vi "test_SegmenterDL100224ThreeD.vi"() -> ()   [LabVIEW 2010, in "SegmenterDL100224ThreeD.lvclass"]
uses:
  SegmenterDL100224ThreeD.lvclass
  common/classes/ImageCollection/ImageCollection/ImageCollection.lvclass
  common/clusters/plugin_specification.ctl
  GenericSegmenter/GenericSegmenter/centroid_cluster.ctl
  <vilib>/vision/Image Controls.llb/IMAQ Image.ctl
  GenericSegmenter/GenericSegmenter/GenericSegmenter.lvclass
  common/classes/GenericComponent/GenericComponent/GenericComponent.lvclass
  common/classes/ImageCollection/ImageCollection/add_mode_enum.ctl
  common/classes/Image/Image/Image.lvclass
panel:
  in  "overlay centroids?":bool
  in  "overlay ROIs?":bool
  out "segmented image":T1(plugin-control)
  in  "segmentButton":bool
  in  "frame":i32(slide) scale=1.0..100.0
  out "original image":T1(plugin-control)
  in  "loadButton":bool
  in  "stopButton":bool
  in  "createButton":bool
  in  "configuration":string(combo)
  # "Test for Segmenter Classes"
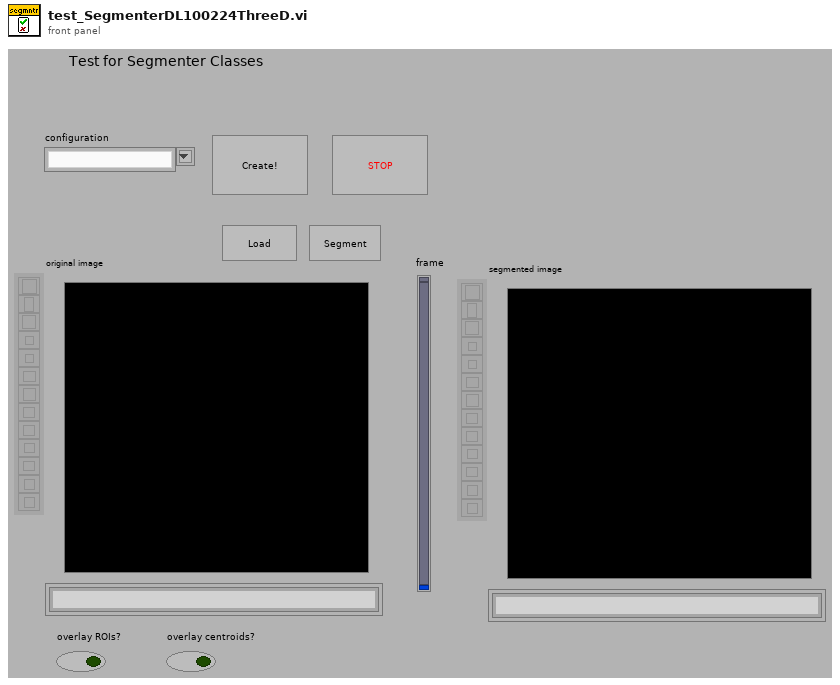
[diagram p1: front panel]
types:
  T1 = typedef "IMAQ Image.ctl" = refnum<image>
  T2 = typedef "GenericSegmenter.lvclass/centroid_cluster.ctl" = cluster{"x":i32, "y":i32, "z":i32, "number of pixels":i32}
  T3 = typedef "plugin_specification.ctl" = cluster{"class path":string, "configuration":string, "label":string, "settings name":string}
  T4 = cluster{"Left":i32, "Top":i32, "Right":i32, "Bottom":i32}
  T5 = typedef "Image Type" = u32
  T6 = typedef "ImageCollection.lvclass/add_mode_enum.ctl" = enum16{"instance", "copy"}
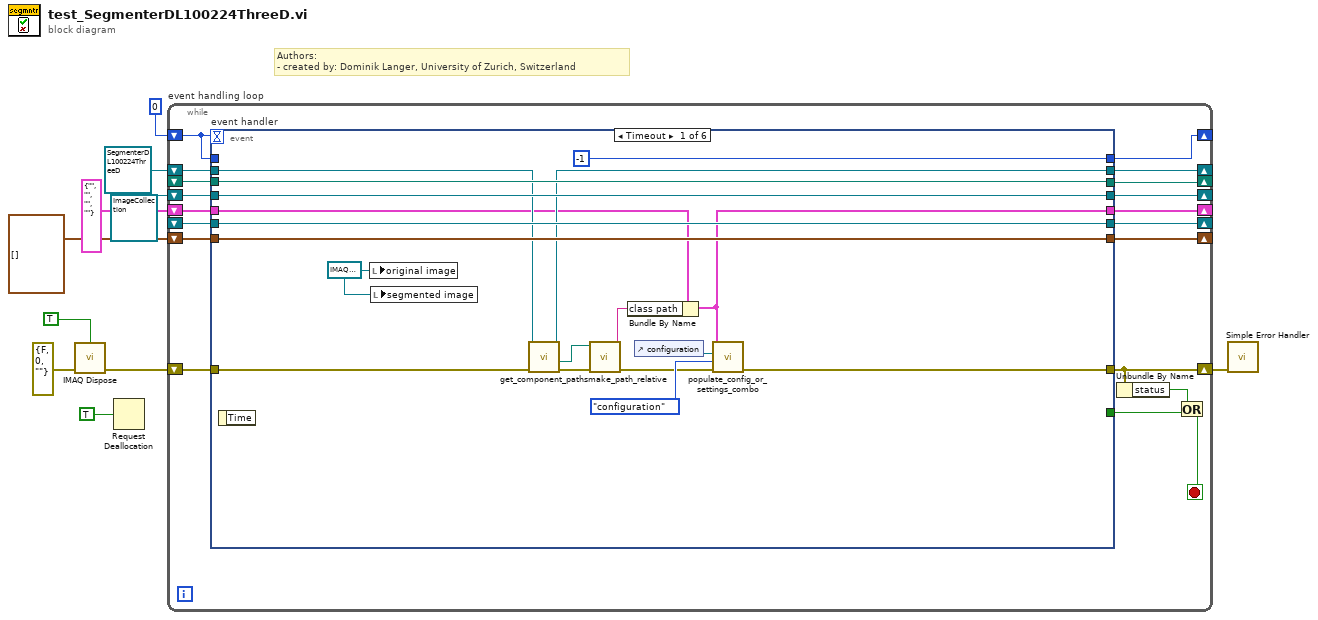
[diagram p0: block diagram]
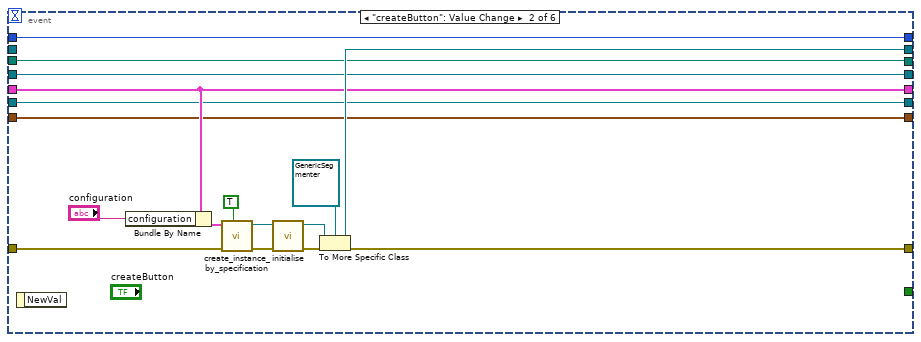
[diagram p2: hidden frame]
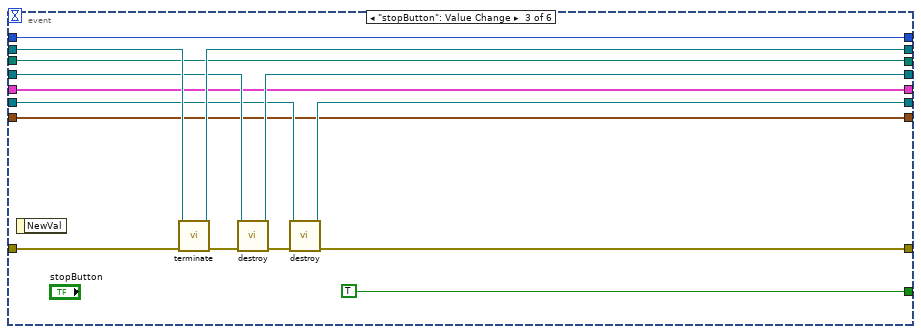
[diagram p3: hidden frame]
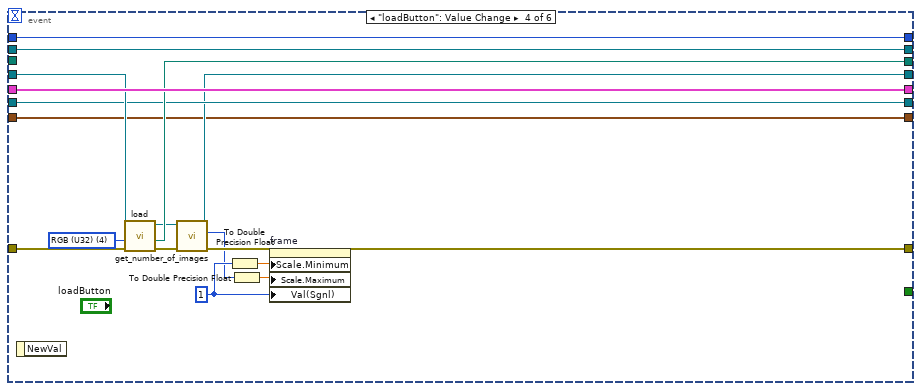
[diagram p4: hidden frame]
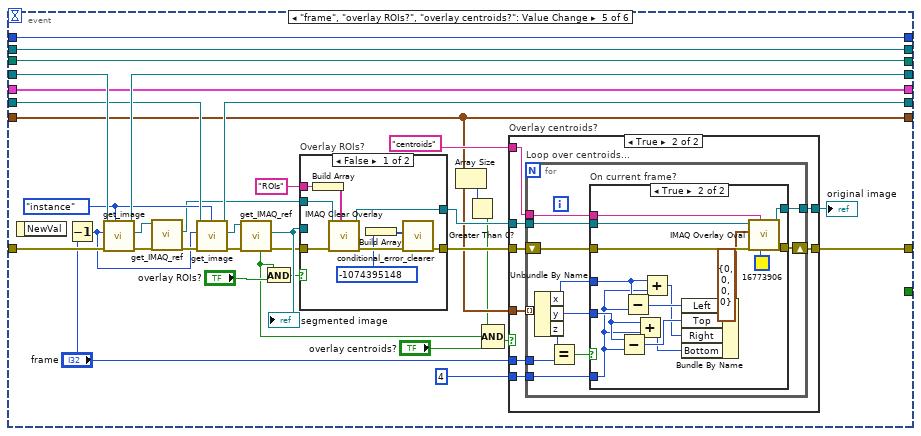
[diagram p5: hidden frame]
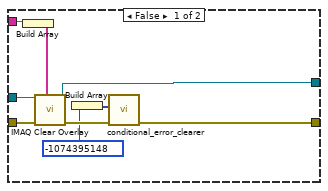
[diagram p6: hidden frame]
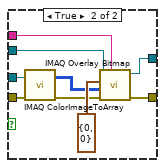
[diagram p8: hidden frame]
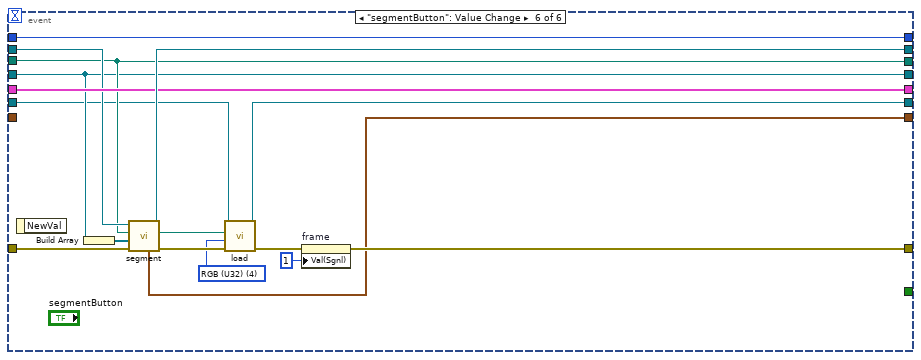
[diagram p9: hidden frame]
diagram:
  # "Authors: \n- created by: Dominik Langer, University of Zurich, Switzerland"
  n1 = call "IMAQ Dispose"("All Images? (No)"=TRUE, "error in (no error)"=errorcluster {"status"=FALSE, "code"=0, "source"=""} ("error out")) -> ("error out"=w4:errorcluster)  [unwired: 4 in]
  n2 = Request Deallocation(TRUE ("flag")) -> ()
  n3 = while "event handling loop" {
    shift-right: [w11] -> w10
    shift-left: w4 -> [w29]
    shift-right: [w25] -> _
    shift-left: refnum<class "SegmenterDL100224ThreeD.lvclass"> refnum ("SegmenterDL100224ThreeD.lvclass") -> [w24]
    shift-right: [w22] -> _
    shift-left: refnum<class "ImageCollection.lvclass"> refnum ("ImageCollection.lvclass") -> [w23]
    shift-right: [w20] -> _
    shift-left: T3 {"class path"="", "configuration"="", "label"="", "settings name"=""} ("component specification") -> [w21]
    shift-right: [w19] -> _
    shift-left: _ -> [w18]
    shift-right: [w16] -> _
    shift-left: 0 -> [w17]
    shift-right: [w15] -> _
    shift-left: _ -> [w14]
    shift-right: [w12] -> _
    shift-left: T2[] [] -> [w13]
    stop <- w26 stop-if-true
    n4 = event "event handler" shown="[0] Timeout" {
      selector: _ -> [_ _ _ _ _ _]
      dyn-events: _ -> [_ _ _ _ _ _]
      timeout: w17 -> [_ _ _ _ _ _]
      tunnel: w29 -> [w36 w64 w78 w92 w131 w211]
      tunnel: [_ _ TRUE _ _ _] -> w27
      tunnel: [w33 w55 w76 w97 w132 w213] -> w25
      tunnel: w24 -> [w34 _ w77 w97 w132 w210]
      tunnel: [w47 w54 w73 w85 w129 w206] -> w22
      tunnel: w23 -> [w47 w54 w74 w91 w130 w206]
      tunnel: w21 -> [w31 w53 w72 w96 w126 w212]
      tunnel: [w30 w53 w72 w96 w126 w212] -> w20
      tunnel: [w46 w51 w71 w94 w125 w209] -> w19
      tunnel: w18 -> [w46 w51 w71 _ w125 w209]
      tunnel: [-1 w50 w70 w95 w124 w208] -> w16
      tunnel: w17 -> [_ w50 w70 w95 w124 w208]
      tunnel: [w43 w49 w68 w89 w122 w204] -> w15
      tunnel: w14 -> [w43 w49 w69 w89 w123 w203]
      tunnel: w13 -> [w42 w48 w65 w80 w103 _]
      tunnel: [w42 w48 w65 w80 w103 w197] -> w12
      tunnel: [w37 w58 w66 w93 w109 w198] -> w11
      event Timeout {
        w44 = T1 refnum ("original image")
        n5 = event-data() -> ()  [unwired: 1 in, 1 out]
        n6 = local write "original image"(w44) -> ()
        n7 = local write "segmented image"(w44) -> ()
        n8 = call-dynamic "get_component_paths.vi"("error in (no error)"=w36, "GenericComponent in"=w34) -> ("error out"=w35:errorcluster, "component class path"=w32:path, "GenericComponent out"=w33:refnum<class "GenericSegmenter.lvclass">)  [unwired: 4 in, 3 out]
        n9 = call "make_path_relative.vi"("error in (no error)"=w35, "absolute path"=w32) -> ("error out"=w39:errorcluster, "relative path"=w38:string)  [unwired: 8 in]
        n10 = Bundle By Name(cluster=w31, "class path"=w38) -> (w30:T3)
        n11 = control-ref of="configuration"() -> (w40:refnum<vi>)
        n12 = call "populate_config_or_settings_combo.vi"("error in (no error)"=w39, "type"=enum16{"configuration", "settings"}."configuration", "combo-box reference"=w40, "plug-in specification"=w30) -> ("error out"=w37:errorcluster)  [unwired: 7 in]
      }
      event "createButton": Value Change {
        n13 = event-data() -> ()  [unwired: 1 in, 1 out]
        n14 = Bundle By Name(cluster=w53, "configuration"="configuration") -> (w62:T3)
        n15 = call "create_instance_by_specification.vi"("call constructor?"=TRUE, "error in (no error)"=w64, "component specification"=w62) -> ("error out"=w61:errorcluster, "GenericPlugin out"=w60:refnum<class "GenericComponent.lvclass">)  [unwired: 6 in, 1 out]
        n16 = call-dynamic "initialise.vi"("error in (no error)"=w61, "GenericPlugin in"=w60) -> ("error out"=w59:errorcluster, "GenericPlugin out"=w57:refnum<class "GenericComponent.lvclass">)  [unwired: 8 in]
        n17 = To More Specific Class(target class=refnum<class "GenericSegmenter.lvclass"> refnum ("GenericSegmenter.lvclass"), reference=w57, error in=w59) -> (specific class reference=w55:refnum<class "GenericSegmenter.lvclass">, error out=w58:errorcluster)
      }
      event "stopButton": Value Change {
        n18 = event-data() -> ()  [unwired: 1 in, 1 out]
        n19 = call-dynamic "terminate.vi"("error in (no error)"=w78, "GenericPlugin in"=w77) -> ("error out"=w75:errorcluster, "GenericPlugin out"=w76:refnum<class "GenericSegmenter.lvclass">)  [unwired: 8 in]
        n20 = call-dynamic "destroy.vi"("error in (no error)"=w75, "ImageCollection in"=w74) -> ("error out"=w67:errorcluster, "ImageCollection out"=w73:refnum<class "ImageCollection.lvclass">)  [unwired: 8 in]
        n21 = call-dynamic "destroy.vi"("error in (no error)"=w67, "ImageCollection in"=w69) -> ("error out"=w66:errorcluster, "ImageCollection out"=w68:refnum<class "ImageCollection.lvclass">)  [unwired: 8 in]
      }
      event "loadButton": Value Change {
        w90 = T5 4 items=["Grayscale (U8)", "Grayscale (I16)", "Grayscale (SGL)", "Complex (CSG)", "RGB (U32)", "HSL (U32)", "RGB (U64)", "Grayscale (U16)"] ("Image Type")
        w83 = 1 ("Value (Signaling)")
        n22 = event-data() -> ()  [unwired: 1 in, 1 out]
        n23 = call "load.vi"("error in (no error)"=w92, "Image Type"=w90, "ImageCollection in"=w91) -> ("error out"=w88:errorcluster, "path out"=w94:path, "ImageCollection out"=w86:refnum<class "ImageCollection.lvclass">)  [unwired: 4 in, 2 out]
        n24 = call-dynamic "get_number_of_images.vi"("error in (no error)"=w88, "ImageCollection in"=w86) -> ("error out"=w87:errorcluster, "size"=w82:i32, "ImageCollection out"=w85:refnum<class "ImageCollection.lvclass">)  [unwired: 7 in]
        n25 = To Double Precision Float(number=w83) -> (double precision float=w84:dbl)
        n26 = To Double Precision Float(number=w82) -> (double precision float=w81:dbl)
        n27 = property on="frame" class="Slide (strict)"(error in=w87, "Scale.Minimum"=w84, "Scale.Maximum"=w81, "Val(Sgnl)"=w83) -> (error out=w93:errorcluster)  [unwired: 1 in, 1 out]
      }
      event "frame", "overlay ROIs?", "overlay centroids?": Value Change {
        w119 = add_mode_enum."instance" ("get image as...")
        n28 = event-data() -> ()  [unwired: 1 in, 1 out]
        n29 = Decrement(x="frame") -> (x-1=w118:i32)
        n30 = call-dynamic "get_image.vi"("get image as..."=w119, "error in (no error)"=w131, "index"=w118, "ImageCollection in"=w130) -> ("error out"=w128:errorcluster, "Image.lvclass"=w127:refnum<class "Image.lvclass">, "ImageCollection out"=w129:refnum<class "ImageCollection.lvclass">)  [unwired: 5 in]
        n31 = call-dynamic "get_IMAQ_ref.vi"("error in (no error)"=w128, "Image.lvclass in"=w127) -> ("error out"=w121:errorcluster, "Image"=w116:T1)  [unwired: 5 in, 3 out]
        n32 = call-dynamic "get_image.vi"("get image as..."=w119, "error in (no error)"=w121, "index"=w118, "ImageCollection in"=w123) -> ("error out"=w117:errorcluster, "Image.lvclass"=w120:refnum<class "Image.lvclass">, "ImageCollection out"=w122:refnum<class "ImageCollection.lvclass">)  [unwired: 5 in]
        n33 = call-dynamic "get_IMAQ_ref.vi"("error in (no error)"=w117, "Image.lvclass in"=w120) -> ("error out"=w114:errorcluster, "Image"=w115:T1, "not empty?"=w100:bool)  [unwired: 5 in, 2 out]
        "segmented image" <- w115
        n34 = And(x=w100, y="overlay ROIs?") -> (x .and. y?=w112:bool)
        n35 = case "Overlay ROIs?" shown="False" w112 {
          tunnel: [w185 w196] -> w108
          tunnel: w116 -> [w186 w195]
          tunnel: w115 -> [_ w191]
          tunnel: w114 -> [w187 w192]
          tunnel: [w181 w193] -> w110
          tunnel: "ROIs" ("Group") -> [w184 w188]
          frame False {
            n36 = Build Array(w184) -> (w183:string[])
            n37 = call "IMAQ Clear Overlay"("Groups"=w183, "error in (no error)"=w187, "Image"=w186) -> ("error out"=w182:errorcluster, "Image Out"=w185:T1)  [unwired: 7 in]
            n38 = Build Array(-1074395148 ("error code")) -> (w180:i32[])
            n39 = call "conditional_error_clearer.vi"("error in (no error)"=w182, "array of clearable error codes"=w180) -> ("error out"=w181:errorcluster)  [unwired: 9 in]
          }
          frame True {
            n40 = call "IMAQ ColorImageToArray"("Image"=w191, "error in (no error)"=w192) -> ("Image Pixels (U32)"=w190:u32[][], "error out"=w189:errorcluster)  [unwired: 2 in, 1 out]
            n41 = call "IMAQ Overlay Bitmap"("Group"=w188, "error in (no error)"=w189, "Bitmap"=w190, "Top Left Point"=cluster{"X":i32, "Y":i32} {"X"=0, "Y"=0}, "Image"=w195) -> ("error out"=w193:errorcluster, "Image Out"=w196:T1)  [unwired: 5 in]
          }
        }
        n42 = Array Size(array=w103) -> (size(s)=w102:i32)
        n43 = Greater Than 0?(x=w102) -> (x > 0?=w98:bool)
        n44 = Compound Arithmetic op=AND(w98, w100, "overlay centroids?") -> (w99:bool)
        n45 = case "Overlay centroids?" shown="True" w99 {
          tunnel: w110 -> [w138 w149]
          tunnel: [w137 w148] -> w109
          tunnel: w103 -> [_ w147]
          tunnel: w108 -> [w134 w146]
          tunnel: "centroids" ("Group") -> [w136 w144]
          tunnel: [w133 w145] -> w106
          tunnel: "frame" -> [_ w143]
          tunnel: 4 -> [_ w142]
          frame False {
            n46 = Build Array(w136) -> (w135:string[])
            n47 = call "IMAQ Clear Overlay"("Groups"=w135, "error in (no error)"=w138, "Image"=w134) -> ("error out"=w141:errorcluster, "Image Out"=w133:T1)  [unwired: 7 in]
            n48 = Build Array(-1074395148 ("error code")) -> (w140:i32[])
            n49 = call "conditional_error_clearer.vi"("error in (no error)"=w141, "array of clearable error codes"=w140) -> ("error out"=w137:errorcluster)  [unwired: 9 in]
          }
          frame True {
            n50 = for "Loop over centroids..." {
              shift-right: [w158] -> w148
              shift-left: w149 -> [w160]
              tunnel: w147 -> [w161] mode=indexing
              tunnel: w146 -> [w159]
              tunnel: [w157] -> w145
              tunnel: w144 -> [w156]
              tunnel: w143 -> [w155]
              tunnel: w142 -> [w150]
              n51 = Unbundle By Name(w161) -> ("x"=w152:i32, "y"=w151:i32, "z"=w154:i32)
              n52 = Equal?(x=w154, y=w155) -> (x = y?=w153:bool)
              n53 = case "On current frame?" shown="True" w153 {
                tunnel: w160 -> [w162 w178]
                tunnel: w159 -> [w163 w177]
                tunnel: [w162 w176] -> w158
                tunnel: [w163 w175] -> w157
                tunnel: w156 -> [_ w174]
                tunnel: w152 -> [_ w171]
                tunnel: w151 -> [_ w172]
                tunnel: w150 -> [_ w170]
                frame False {
                }
                frame True {
                  n54 = Subtract(x=w172, y=w170) -> (x-y=w167:i32)
                  n55 = Subtract(x=w171, y=w170) -> (x-y=w168:i32)
                  n56 = Add(x=w172, y=w170) -> (x+y=w165:i32)
                  n57 = Add(x=w171, y=w170) -> (x+y=w166:i32)
                  n58 = Bundle By Name(cluster=T4 {"Left"=0, "Top"=0, "Right"=0, "Bottom"=0} ("Bounding Rectangle"), "Left"=w168, "Top"=w167, "Right"=w166, "Bottom"=w165) -> (w164:T4)
                  n59 = call "IMAQ Overlay Oval"("Color"=u32 16773906, "Group"=w174, "error in (no error)"=w178, "Bounding Rectangle"=w164, "Image"=w177) -> ("error out"=w176:errorcluster, "Image Out"=w175:T1)  [unwired: 5 in]
                }
              }
            }
          }
        }
        "original image" <- w106
      }
      event "segmentButton": Value Change {
        w201 = T5 4 items=["Grayscale (U8)", "Grayscale (I16)", "Grayscale (SGL)", "Complex (CSG)", "RGB (U32)", "HSL (U32)", "RGB (U64)", "Grayscale (U16)"] ("Image Type")
        n60 = event-data() -> ()  [unwired: 1 in, 1 out]
        n61 = Build Array(w206) -> (w207:refnum<class "ImageCollection.lvclass">[])
        n62 = call-dynamic "segment.vi"("error in (no error)"=w211, "ImageCollection in"=w207, "image file path"=w209, "GenericSegmenter in"=w210) -> ("error out"=w205:errorcluster, "segmented image path out"=w202:path, "GenericSegmenter out"=w213:refnum<class "GenericSegmenter.lvclass">, "centroids"=w197:T2[])  [unwired: 3 in, 1 out]
        n63 = call "load.vi"("error in (no error)"=w205, "Image Type"=w201, "path in"=w202, "ImageCollection in"=w203) -> ("error out"=w200:errorcluster, "ImageCollection out"=w204:refnum<class "ImageCollection.lvclass">)  [unwired: 3 in, 3 out]
        n64 = property on="frame" class="Slide (strict)"(error in=w200, "Val(Sgnl)"=1 ("Value (Signaling)")) -> (error out=w198:errorcluster)  [unwired: 1 in, 1 out]
      }
    }
    n65 = Unbundle By Name(w11) -> ("status"=w28:bool)
    n66 = Or(x=w28, y=w27) -> (x .or. y?=w26:bool)
  }
  n67 = call <vilib>:"Simple Error Handler.vi"("error in (no error)"=w10) -> ()  [unwired: 4 in, 5 out]
